vi "Generate Scan List.vi"(10 "Panel":enum16{"Panel 1", "Panel 2", "Panel 3"}(ring), 11 "Panel":T1[][](array[typedef])) -> (1 "Panel List":string[](array[string]), 2 "Channel Number":string[](array[string]), 3 "Channel Label":string[](array[string]))   [LabVIEW 2013]
uses:
  Type Definitions/Channel Label.ctl
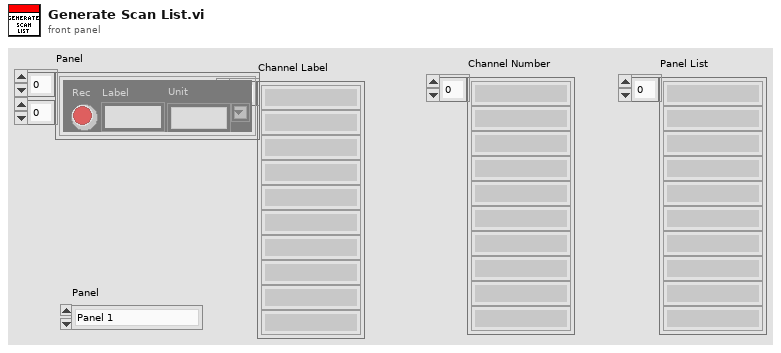
[diagram p1: front panel]
types:
  T1 = typedef "Channel Label.ctl" = cluster{"Label":string, "Chan":string, "Rec":bool, "Unit":string}
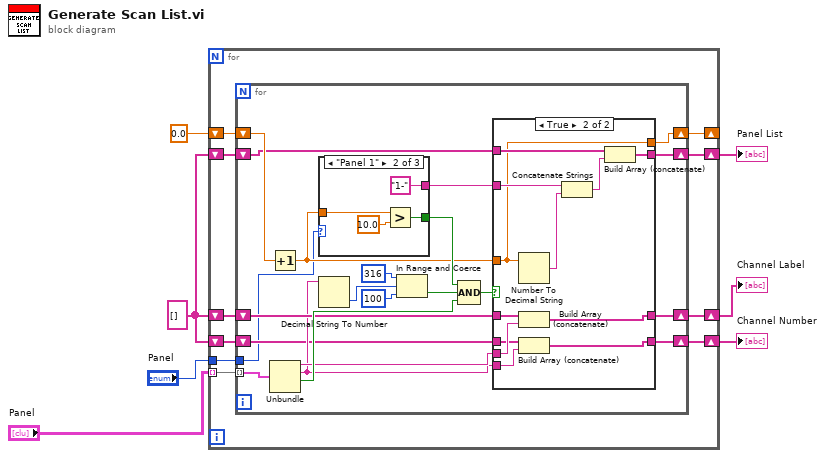
[diagram p0: block diagram]
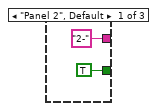
[diagram p2: hidden frame]
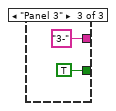
[diagram p3: hidden frame]
diagram:
  w7 = string[] []
  n1 = for {
    tunnel: "Panel" -> [w17] mode=indexing
    shift-right: [w16] -> w2
    shift-left: w7 -> [w15]
    shift-right: [w14] -> w1
    shift-left: w7 -> [w13]
    shift-right: [w11] -> _
    shift-left: 0.0 -> [w12]
    shift-right: [w9] -> w3
    shift-left: w7 -> [w10]
    tunnel: "Panel" -> [w8]
    n2 = for {
      tunnel: w17 -> [w38] mode=indexing
      shift-right: [w30] -> w16
      shift-left: w15 -> [w24]
      shift-right: [w20] -> w14
      shift-left: w13 -> [w21]
      shift-right: [w29] -> w11
      shift-left: w12 -> [w32]
      shift-right: [w26] -> w9
      shift-left: w10 -> [w27]
      tunnel: w8 -> [w19]
      n3 = Increment(x=w32) -> (x+1=w28:dbl)
      n4 = Unbundle(w38) -> ("Label"=w23:string, "Chan"=w22:string, "Rec"=w33:bool)  [unwired: 1 out]
      n5 = case shown="\"Panel 1\"" w19 {
        tunnel: [TRUE w43 TRUE] -> w31
        tunnel: w28 -> [_ w42 _]
        tunnel: ["2-" "1-" "3-"] -> w18
        frame "Panel 2", Default {
        }
        frame "Panel 1" {
          n6 = Greater?(x=w42, y=10.0) -> (0:w43:bool)
        }
        frame "Panel 3" {
        }
      }
      n7 = Decimal String To Number(string=w22) -> (number=w37:i32)  [unwired: 2 in, 1 out]
      n8 = In Range and Coerce(upper limit=316, x=w37, lower limit=100) -> (In Range?=w34:bool)  [unwired: 1 out]
      n9 = Compound Arithmetic op=AND(w31, w34, w33) -> (w25:bool)
      n10 = case shown="True" w25 {
        tunnel: w23 -> [_ w62]
        tunnel: [w50 w61] -> w30
        tunnel: w24 -> [w50 w59]
        tunnel: [w47 w60] -> w20
        tunnel: w22 -> [_ w58]
        tunnel: w21 -> [w47 w57]
        tunnel: w28 -> [w49 w51]
        tunnel: [w48 w56] -> w26
        tunnel: [w49 w51] -> w29
        tunnel: w18 -> [_ w55]
        tunnel: w27 -> [w48 w52]
        frame False {
        }
        frame True {
          n11 = Number To Decimal String(number=w51) -> (decimal integer string=w54:string)  [unwired: 1 in]
          n12 = Build Array (concatenate)(w59, w62) -> (w61:string[])
          n13 = Build Array (concatenate)(w57, w58) -> (w60:string[])
          n14 = Concatenate Strings(w55, w54) -> (w53:string)
          n15 = Build Array (concatenate)(w52, w53) -> (w56:string[])
        }
      }
    }
  }
  "Panel List" <- w3
  "Channel Number" <- w1
  "Channel Label" <- w2
